vi "Mechanical Action.vi"() -> ()   [LabVIEW 2023]
doc: "This VI demonstrates the mechanical action of Boolean controls. The light turns on and the counter increments when a button's value is true. The light turns off and the counter stays the same when a button's value is false. The default state for all the buttons is false.\n\nThere are two kinds of Boolean mechanical action: switch and latch. Switch will return to its default state when directed by the user. Latch will return to its default state when directed by the user or when its value has been read from the terminal on the block diagram."
panel:
  in  "Mechanical Actions":T1(radio)
  out "Tab Control":T1(tab)
  in  "switch when pressed button":bool
  out "switch when pressed status":bool
  out "switch when pressed counter":i32
  in  "switch when released button":bool
  out "switch when released status":bool
  out "switch when released counter":i32
  in  "switch until released button":bool
  out "switch until released status":bool
  out "switch until released counter":i32
  in  "latch when pressed button":bool
  out "latch when pressed status":bool
  out "latch when pressed counter":i32
  in  "latch when released button":bool
  out "latch when released status":bool
  out "latch when released counter":i32
  in  "latch until released button":bool
  out "latch until released counter":i32
  out "latch until released status":bool
  in  "Clear Counters":bool
  in  "Stop":bool
  # "Overview: Demonstrates the different Mechanical Action settings of Boolean controls.\nInstructions:\n1. Run the VI.\n2. Select a picture in the Mechanical Actions control.\n3. Click and hold the corresponding button to demonstrate the control operation for the selected mechanical action.\n4. Repeat steps 2 and 3 for the other selections in the Mechanical Actions control.\n5. Click Stop to stop the VI."
  # "The arrangement of these options corresponds to the selections in the Mechanical Action right-click menu for Boolean controls."
  # "Boolean controls can have one of six possible Mechanical Action settings. The status light turns on and the counter increments when a button's value is true. The default state for all the buttons is false. There are two categories of mechanical action: switch and latch. Switch will return to its default state when directed by the user. Latch will return to its default state when directed by the user or when its value has been read from the terminal on the block diagram."
  # "Switch When Pressed - Change state on a button press.  Remain there until another button press."
  # "Switch When Released - Change state on a button release.  Remain there until another button release."
  # "Switch Until Released - Change state on a button press.  Change back when the button is released."
  # "Latch When Pressed - Change state on a button press.  Change back when the control is read by LabVIEW."
  # "Latch When Released - Change state on a button release. Change back when the control is read by LabVIEW."
  # "Latch Until Released - Change state on a button press. Change back when released and read by LabVIEW."
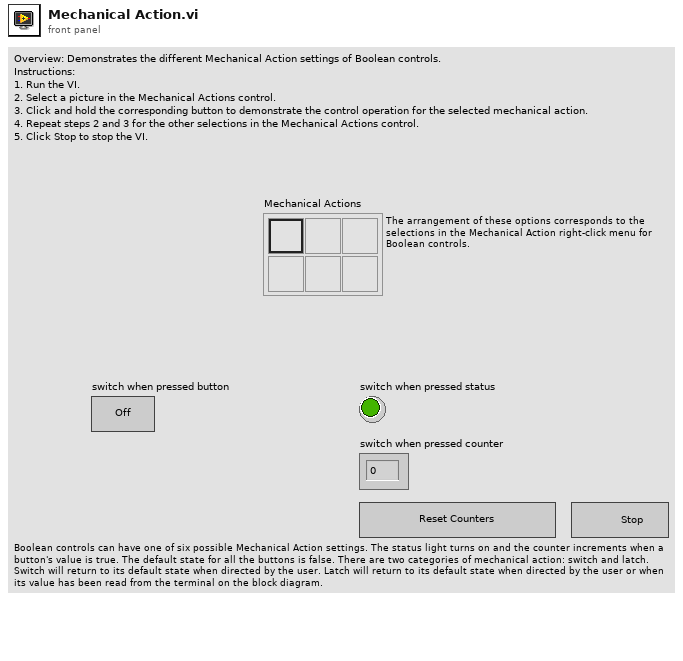
[diagram p1: front panel]
types:
  T1 = enum32{"Switch When Pressed", "Switch When Released", "Switch Until Released", "Latch When Pressed", "Latch When Released", "Latch Until Released"}
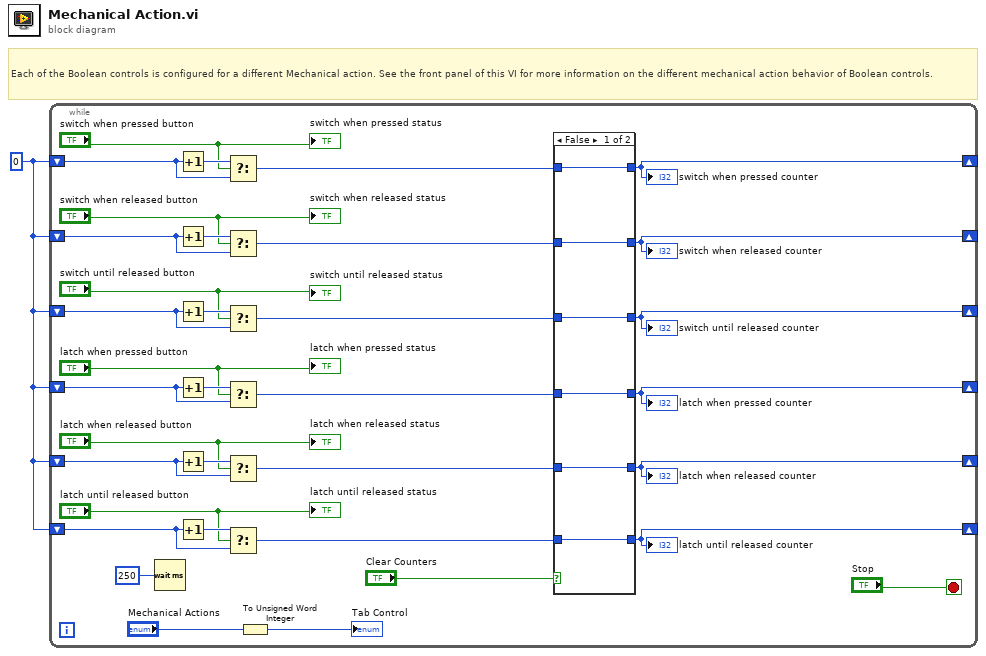
[diagram p0: block diagram]
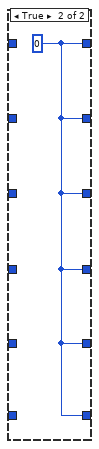
[diagram p2: hidden frame]
diagram:
  w1 = 0
  # "Each of the Boolean controls is configured for a different Mechanical action. See the front panel of this VI for more information on the different mechanical action behavior of Boolean controls."
  n1 = while {
    shift-left: w1 -> [w25]
    shift-right: [w12] -> _
    shift-left: w1 -> [w28]
    shift-right: [w11] -> _
    shift-left: w1 -> [w29]
    shift-right: [w10] -> _
    shift-left: w1 -> [w32]
    shift-right: [w9] -> _
    shift-left: w1 -> [w33]
    shift-right: [w8] -> _
    shift-left: w1 -> [w35]
    shift-right: [w7] -> _
    stop <- "Stop" stop-if-true
    n2 = Wait (ms)(milliseconds to wait=u32 250) -> ()  [unwired: 1 out]
    n3 = Increment(x=w25) -> (x+1=w26:i32)
    n4 = Increment(x=w28) -> (x+1=w27:i32)
    n5 = Increment(x=w29) -> (x+1=w30:i32)
    n6 = Increment(x=w32) -> (x+1=w31:i32)
    n7 = Increment(x=w33) -> (x+1=w34:i32)
    n8 = Increment(x=w35) -> (x+1=w36:i32)
    n9 = Select(t=w26, s="switch when pressed button", f=w25) -> (s? t:f=w19:i32)
    n10 = Select(t=w27, s="switch when released button", f=w28) -> (s? t:f=w20:i32)
    n11 = Select(t=w30, s="switch until released button", f=w29) -> (s? t:f=w21:i32)
    n12 = Select(t=w31, s="latch when pressed button", f=w32) -> (s? t:f=w22:i32)
    n13 = Select(t=w34, s="latch when released button", f=w33) -> (s? t:f=w23:i32)
    n14 = Select(t=w36, s="latch until released button", f=w35) -> (s? t:f=w24:i32)
    n15 = To Unsigned Word Integer(number="Mechanical Actions") -> (unsigned 16bit integer=→"Tab Control":u16)
    n16 = case shown="False" "Clear Counters" {
      tunnel: [w42 w43] -> w7
      tunnel: w24 -> [w42 _]
      tunnel: [w41 w43] -> w8
      tunnel: w23 -> [w41 _]
      tunnel: [w40 w43] -> w9
      tunnel: w22 -> [w40 _]
      tunnel: [w39 w43] -> w10
      tunnel: w21 -> [w39 _]
      tunnel: [w38 w43] -> w11
      tunnel: w20 -> [w38 _]
      tunnel: [w37 w43] -> w12
      tunnel: w19 -> [w37 _]
      frame False {
      }
      frame True {
        w43 = 0
      }
    }
    "switch when pressed counter" <- w12
    "switch when released counter" <- w11
    "switch until released counter" <- w10
    "latch when pressed counter" <- w9
    "latch when released counter" <- w8
    "latch until released counter" <- w7
    "switch when pressed status" <- "switch when pressed button"
    "switch when released status" <- "switch when released button"
    "switch until released status" <- "switch until released button"
    "latch when pressed status" <- "latch when pressed button"
    "latch when released status" <- "latch when released button"
    "latch until released status" <- "latch until released button"
  }
